vi "POI to NormPOI.vi"(0 "X start":dbl, 1 "FrameSize":dbl, 2 "Zoom":dbl, 5 "Y start":dbl, 7 "Z start":dbl, 9 "X stop":dbl, 12 "Y stop":dbl, 14 "Z stop":dbl) -> (3 "Norm XStart":dbl, 4 "Norm YStart":dbl, 6 "Norm ZStart":dbl, 8 "Norm XStop":dbl, 10 "Norm YStop":dbl, 15 "Norm ZStop":dbl)   [LabVIEW 2017]
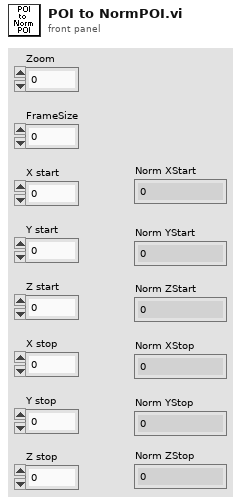
[diagram p1: front panel]
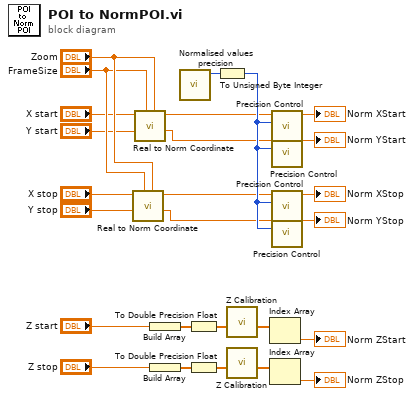
[diagram p0: block diagram]
diagram:
  n1 = call "Real to Norm Coordinate.vi"("Zoom"="Zoom", "FrameSize"="FrameSize", "Y"="Y stop", "X"="X stop") -> ("Norm. Y"=w22:dbl, "Norm. X"=w20:dbl)  [unwired: 6 in]
  n2 = call "Real to Norm Coordinate.vi"("Zoom"="Zoom", "FrameSize"="FrameSize", "Y"="Y start", "X"="X start") -> ("Norm. Y"=w18:dbl, "Norm. X"=w16:dbl)  [unwired: 6 in]
  n3 = Build Array("Z start") -> (w9:dbl[])
  n4 = Build Array("Z stop") -> (w12:dbl[])
  n5 = call "Normalised values precision.vi"() -> ("Normalised values precision"=w3:i32)  [unwired: 11 in]
  n6 = To Double Precision Float(number=w9) -> (double precision float=w15:dbl[])
  n7 = To Double Precision Float(number=w12) -> (double precision float=w14:dbl[])
  n8 = To Unsigned Byte Integer(number=w3) -> (unsigned 8bit integer=w24:u8)
  n9 = call "Z Calibration.vi"("Z Planes"=w15) -> ("Norm Z"=w10:dbl[])  [unwired: 7 in, 3 out]
  n10 = call "Z Calibration.vi"("Z Planes"=w14) -> ("Norm Z"=w11:dbl[])  [unwired: 7 in, 3 out]
  n11 = Index Array(array=w10) -> (element=→"Norm ZStart":dbl)  [unwired: 1 in]
  n12 = Index Array(array=w11) -> (element=→"Norm ZStop":dbl)  [unwired: 1 in]
  n13 = call <userlib>:"Precision Control.vi"("Precision"=w24, "Input Value"=w16) -> ("Output Value"=→"Norm XStart":dbl)  [unwired: 8 in, 1 out]
  n14 = call <userlib>:"Precision Control.vi"("Precision"=w24, "Input Value"=w18) -> ("Output Value"=→"Norm YStart":dbl)  [unwired: 8 in, 1 out]
  n15 = call <userlib>:"Precision Control.vi"("Precision"=w24, "Input Value"=w20) -> ("Output Value"=→"Norm XStop":dbl)  [unwired: 8 in, 1 out]
  n16 = call <userlib>:"Precision Control.vi"("Precision"=w24, "Input Value"=w22) -> ("Output Value"=→"Norm YStop":dbl)  [unwired: 8 in, 1 out]
